vi "Motor_Limit.vi"(0 "Current_Pos":dbl, 1 "Motor_Speed":dbl, 2 "Scale Positions":T1) -> (14 "New_Motor_Speed":dbl, 15 "At Limit":bool)   [LabVIEW 2016, in "ArgosLib.lvlib"]
uses:
  TypeDefs/MotorLimitPositions_Type.ctl
  ArgosLib.lvlib
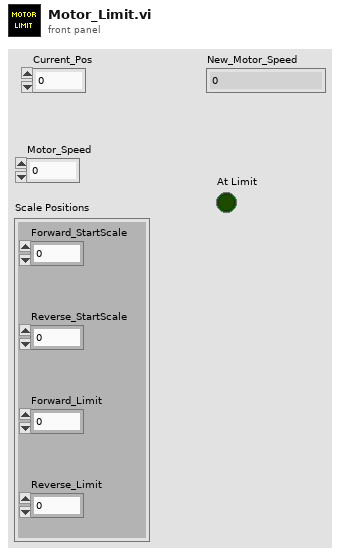
[diagram p1: front panel]
types:
  T1 = typedef "MotorLimitPositions_Type.ctl" = cluster{"Forward_StartScale":dbl, "Reverse_StartScale":dbl, "Forward_Limit":dbl, "Reverse_Limit":dbl}
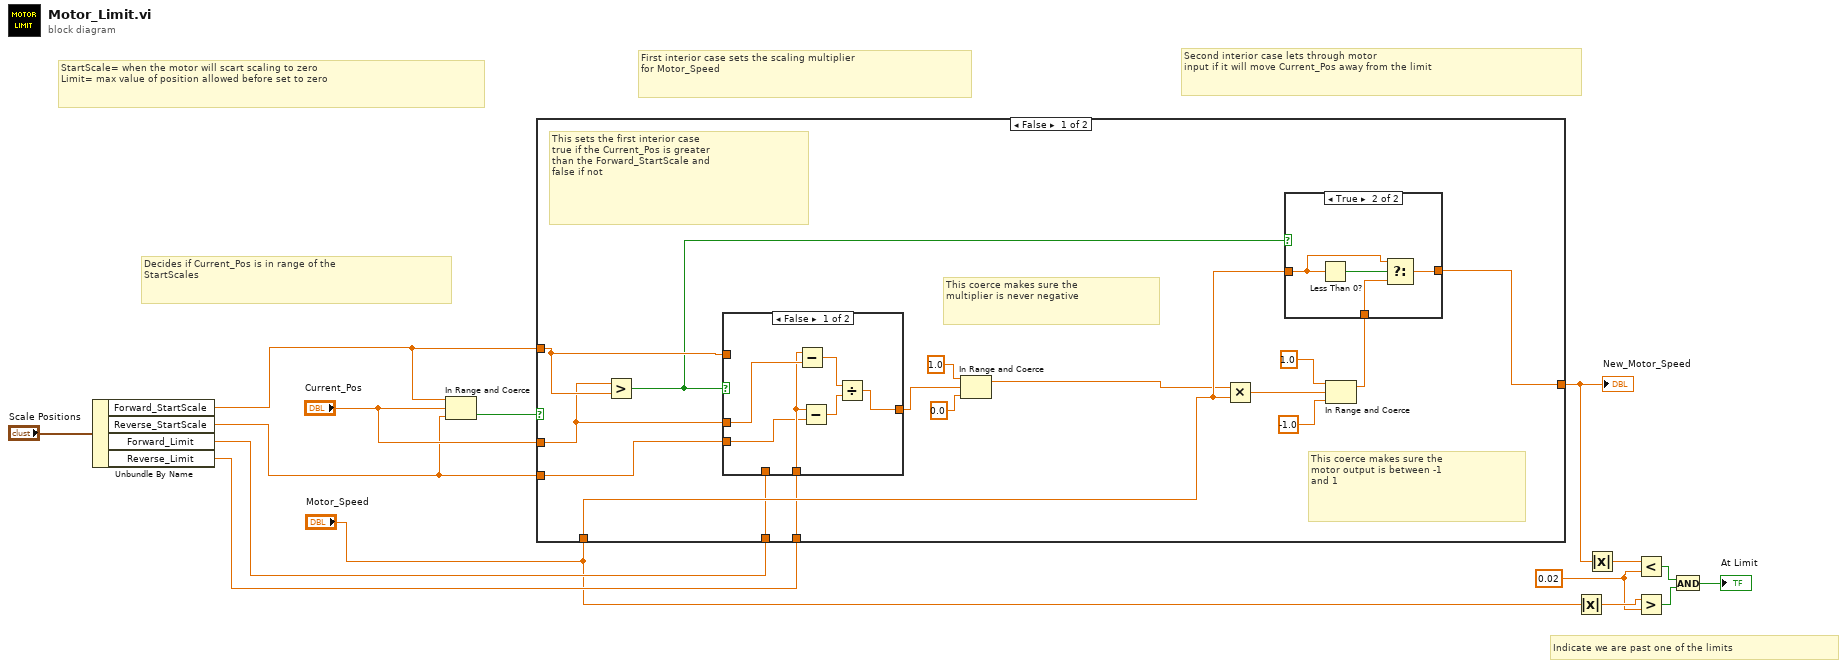
[diagram p0: block diagram]
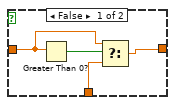
[diagram p2: hidden frame]
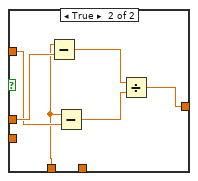
[diagram p3: hidden frame]
diagram:
  w1 = 0.02 ("y")
  # "Indicate we are past one of the limits"
  # "Second interior case lets through motor \ninput if it will move Current_Pos away from the limit"
  # "First interior case sets the scaling multiplier\nfor Motor_Speed"
  # "Decides if Current_Pos is in range of the\nStartScales"
  # "StartScale= when the motor will scart scaling to zero\nLimit= max value of position allowed before set to zero"
  n1 = Unbundle By Name("Scale Positions") -> ("Forward_StartScale"=w12:dbl, "Reverse_StartScale"=w11:dbl, "Forward_Limit"=w10:dbl, "Reverse_Limit"=w9:dbl)
  n2 = In Range and Coerce(upper limit=w12, x="Current_Pos", lower limit=w11) -> (In Range?=w15:bool)  [unwired: 1 out]
  n3 = case shown="False" w15 {
    tunnel: "Motor_Speed" -> [w25 w52]
    tunnel: [w16 w52] -> w8
    tunnel: "Current_Pos" -> [w23 _]
    tunnel: w12 -> [w30 _]
    tunnel: w11 -> [w31 _]
    tunnel: w10 -> [w21 _]
    tunnel: w9 -> [w22 _]
    frame False {
      # "This coerce makes sure the \nmotor output is between -1\nand 1"
      # "This coerce makes sure the\nmultiplier is never negative"
      # "This sets the first interior case\ntrue if the Current_Pos is greater \nthan the Forward_StartScale and\nfalse if not"
      n4 = Greater?(x=w23, y=w30) -> (0:w26:bool)
      n5 = case shown="False" w26 {
        tunnel: w31 -> [w40 _]
        tunnel: w30 -> [_ w50]
        tunnel: w23 -> [w44 w51]
        tunnel: w21 -> [_ w49]
        tunnel: w22 -> [w41 _]
        tunnel: [w45 w46] -> w20
        frame False {
          n6 = Subtract(x=w41, y=w44) -> (x-y=w43:dbl)
          n7 = Subtract(x=w41, y=w40) -> (x-y=w42:dbl)
          n8 = Divide(x=w43, y=w42) -> (x/y=w45:dbl)
        }
        frame True {
          n9 = Subtract(x=w49, y=w51) -> (x-y=w48:dbl)
          n10 = Subtract(x=w49, y=w50) -> (x-y=w47:dbl)
          n11 = Divide(x=w48, y=w47) -> (x/y=w46:dbl)
        }
      }
      n12 = In Range and Coerce(upper limit=1.0, x=w20, lower limit=0.0) -> (coerced(x)=w17:dbl)  [unwired: 1 out]
      n13 = Multiply(x=w17, y=w25) -> (x*y=w27:dbl)
      n14 = In Range and Coerce(upper limit=1.0, x=w27, lower limit=-1.0) -> (coerced(x)=w24:dbl)  [unwired: 1 out]
      n15 = case shown="True" w26 {
        tunnel: w25 -> [w32 w38]
        tunnel: w24 -> [w33 w37]
        tunnel: [w35 w36] -> w16
        frame False {
          n16 = Greater Than 0?(x=w32) -> (x > 0?=w34:bool)
          n17 = Select(t=w32, s=w34, f=w33) -> (s? t:f=w35:dbl)
        }
        frame True {
          n18 = Less Than 0?(x=w38) -> (x < 0?=w39:bool)
          n19 = Select(t=w38, s=w39, f=w37) -> (s? t:f=w36:dbl)
        }
      }
    }
    frame True {
      # "Passes through Motor_Speed if \nCurrent_Pos is in range"
    }
  }
  "New_Motor_Speed" <- w8
  n20 = Absolute Value(x="Motor_Speed") -> (abs(x)=w2:dbl)
  n21 = Absolute Value(x=w8) -> (abs(x)=w3:dbl)
  n22 = Less?(x=w3, y=w1) -> (x < y?=w6:bool)
  n23 = Greater?(x=w2, y=w1) -> (0:w5:bool)
  n24 = And(x=w6, y=w5) -> (x .and. y?=→"At Limit":bool)
